vi "Fill Employee Info Data Set.vi"(8 "error in (no error)":errorcluster caption="错误输入（无错误）", 11 "Employee 输入":refnum<class "Employee.lvclass"> caption="DNL_LabVIEW Object in") -> (0 "error out":errorcluster caption="错误输出", 3 "Employee 输出":refnum<class "Employee.lvclass"> caption="DNL_LabVIEW Object out")   [LabVIEW 2012, in "Employee.lvclass"]
uses:
  Employee.lvclass
  Employee.lvclass/Employee.ctl
  Data Set/DataSet.lvclass
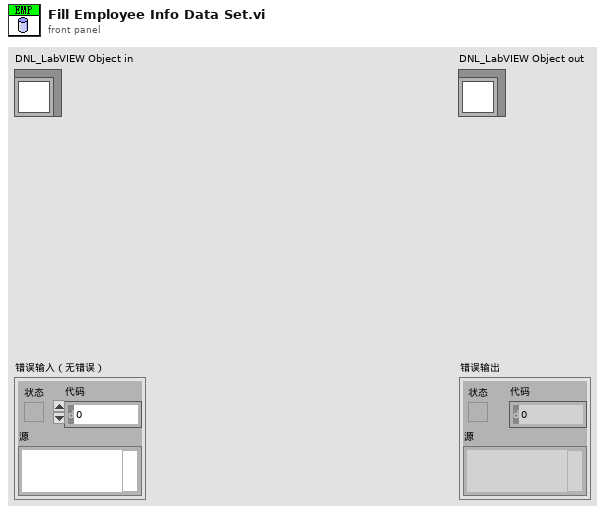
[diagram p1: front panel]
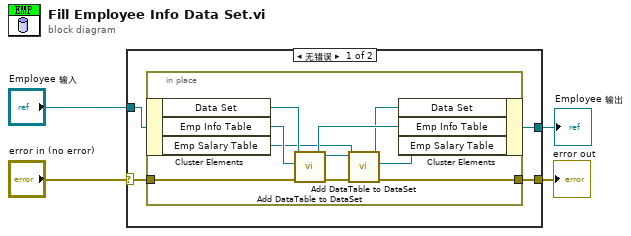
[diagram p0: block diagram]
diagram:
  n1 = case shown="无错误" "error in (no error)" {
    selector: "error in (no error)" -> [w7 w20]
    tunnel: [w5 w20] -> w3
    tunnel: [w6 w19] -> w2
    tunnel: "Employee 输入" -> [w8 w19]
    frame No Error {
      n2 = in-place {
        in-place-border: w7 -> [w17]
        in-place-border: [w9] -> w5
        n3 = in-place-cluster #1(w8) -> ("Data Set"=w18:refnum<class "DataSet.lvclass">, "Emp Info Table"=w16:refnum<class "DataTable.lvclass">, "Emp Salary Table"=w12:refnum<class "DataTable.lvclass">)
        n4 = call "Add DataTable to DataSet.vi"("error in (no error)"=w17, "Data Grid VIEW.lvlib:DataTable.lvclass"=w16, "DataSet 输入"=w18) -> ("error out"=w14:errorcluster, "DataTable输出"=w15:refnum<class "DataTable.lvclass">, "DataSet 输出"=w13:refnum<class "DataSet.lvclass">)  [unwired: 6 in]
        n5 = call "Add DataTable to DataSet.vi"("error in (no error)"=w14, "Data Grid VIEW.lvlib:DataTable.lvclass"=w12, "DataSet 输入"=w13) -> ("error out"=w9:errorcluster, "DataTable输出"=w11:refnum<class "DataTable.lvclass">, "DataSet 输出"=w10:refnum<class "DataSet.lvclass">)  [unwired: 6 in]
        n6 = in-place-cluster #1("Data Set"=w10, "Emp Info Table"=w15, "Emp Salary Table"=w11) -> (w6:refnum<class "Employee.lvclass">)
      }
    }
    frame Error {
    }
  }
  "error out" <- w3
  "Employee 输出" <- w2
